vi "Initialize Parameters.vi"(8 "error in (no error)":errorcluster, 10 "Cluster":T1={"Save Options"={"Primary Storage Location"=path "", "Backup Storage Location"=path "", "Enable Primary"=FALSE, "Enable Secondary"=FALSE, "Save Image as"=enum."RAW"}, "Other Settings"={"Show Image Averaging Option"=TRUE, "Component Name Prefix"=""}, "PLC Parameters"={"Initialize Parameters"={"VISA  Port"="", "Baud Rate"=0}, "Wakeup Bit (Set)"={"Address"=0, "Set/Reset"=FALSE}, "Incoming Bit (Get)"={"Address"=0, "Set/Reset"=FALSE}, "Acknowledge Bit (Set)"={"Address"=0, "Set/Reset"=FALSE}}}, 11 "Controller in":refnum<class "Controller.lvclass">) -> (0 "error out":errorcluster, 3 "Controller out":refnum<class "Controller.lvclass">)   [LabVIEW 2022 SP3, in "Controller.lvlib" / "Controller.lvclass"]
uses:
  Controller.lvclass
  Controller.lvclass/Controller.ctl
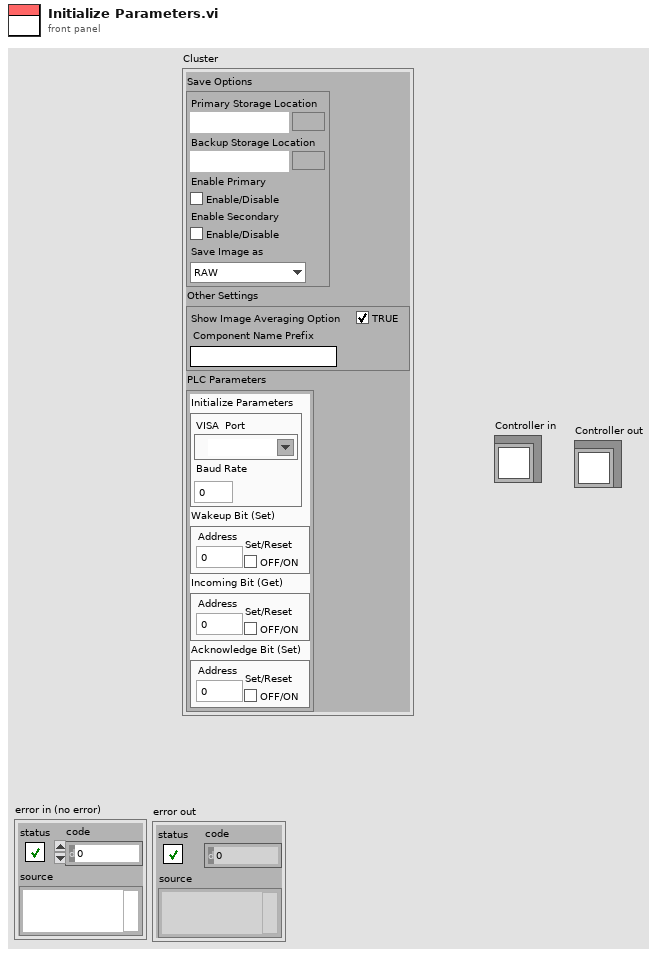
[diagram p1: front panel]
types:
  T1 = cluster{"Save Options":cluster{"Primary Storage Location":path, "Backup Storage Location":path, "Enable Primary":bool, "Enable Secondary":bool, "Save Image as":enum16{"RAW", "TIFF"}}, "Other Settings":cluster{"Show Image Averaging Option":bool, "Component Name Prefix":string}, "PLC Parameters":cluster{"Initialize Parameters":cluster{"VISA  Port":refnum<visa-resource-name>, "Baud Rate":u32}, "Wakeup Bit (Set)":cluster{"Address":u16, "Set/Reset":bool}, "Incoming Bit (Get)":cluster{"Address":u16, "Set/Reset":bool}, "Acknowledge Bit (Set)":cluster{"Address":u16, "Set/Reset":bool}}}
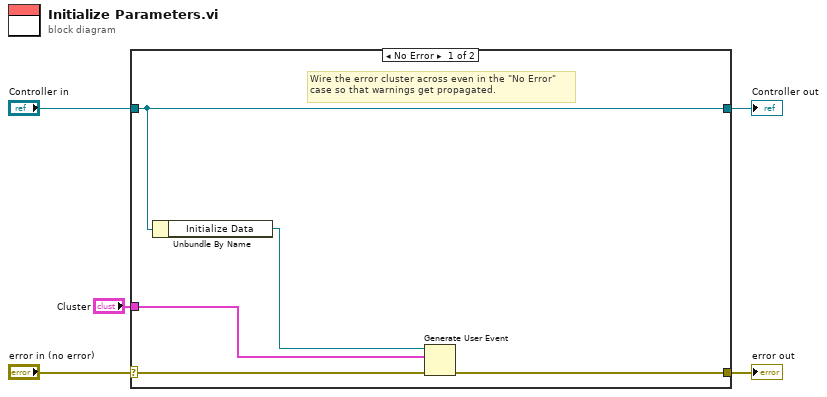
[diagram p0: block diagram]
diagram:
  n1 = case shown="No Error" "error in (no error)" {
    selector: "error in (no error)" -> [w7 w12]
    tunnel: [w6 w12] -> w4
    tunnel: [w9 w11] -> w2
    tunnel: "Controller in" -> [w9 w11]
    tunnel: "Cluster" -> [w10 _]
    frame No Error {
      # "Wire the error cluster across even in the \"No Error\"\ncase so that warnings get propagated."
      n2 = Unbundle By Name(w9) -> ("Initialize Data"=w8:refnum<user-event>)
      n3 = Generate User Event(user event=w8, event data cluster=w10, error in=w7) -> (error out=w6:errorcluster)  [unwired: 1 in, 1 out]
    }
    frame Error {
    }
  }
  "error out" <- w4
  "Controller out" <- w2
